vi "FusePose.vi"(0 "LIDAR range deltaX":dbl, 1 "LIDAR range deltaY":dbl, 2 "LimeLight PnP deltaX":dbl, 3 "LimeLight PnP deltaY":dbl, 4 "LimeLight range deltaX":dbl, 5 "LimeLight range deltaY":dbl, 6 "Odometry deltaY":dbl, 8 "Odometry deltaX":dbl) -> (14 "Fused deltaX":dbl, 19 "Fused deltaY":dbl)   [LabVIEW 2019]
doc: "This VI fuses multiple sensing modalities to estimate the robot's current pose."
uses:
  <vilib>/Rock Robotics/WPI/DriverStation/WPI_DriverStationRobotMode2.ctl
  sensors.vi
  dsdata.vi
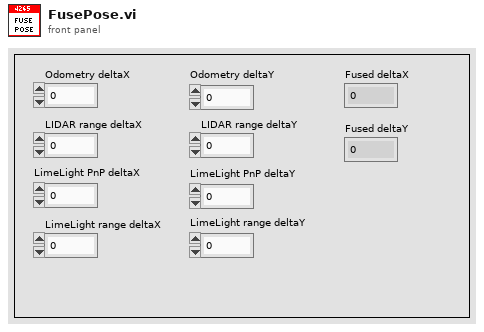
[diagram p1: front panel]
types:
  T1 = typedef "WPI_DriverStationRobotMode2.ctl" = enum16{"Autonomous Disabled", "Autonomous Enabled", "Teleop Disabled", "Teleop Enabled", "Disconnected", "Finish", "Test Disabled", "Test Enabled", "Emergency Stopped"}
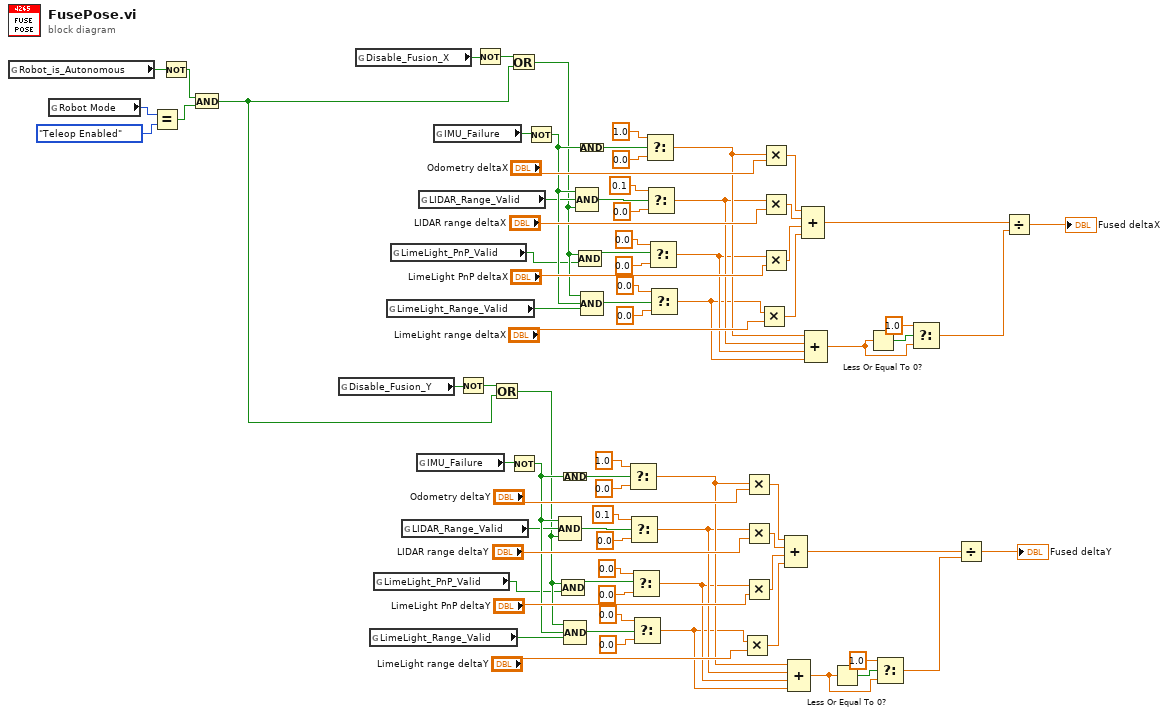
[diagram p0: block diagram]
diagram:
  n1 = global read "dsdata.vi" "Robot_is_Autonomous"() -> (w55:bool)
  n2 = global read "dsdata.vi" "Robot Mode"() -> (w54:T1)
  n3 = Equal?(x=w54, y=WPI_DriverStationRobotMode2."Teleop Enabled") -> (x = y?=w53:bool)
  n4 = Not(x=w55) -> (.not. x?=w52:bool)
  n5 = And(x=w52, y=w53) -> (x .and. y?=w9:bool)
  n6 = global read "dsdata.vi" "Disable_Fusion_Y"() -> (w16:bool)
  n7 = global read "dsdata.vi" "Disable_Fusion_X"() -> (w50:bool)
  n8 = global read "sensors.vi" "LimeLight_Range_Valid"() -> (w11:bool)
  n9 = global read "sensors.vi" "LimeLight_PnP_Valid"() -> (w12:bool)
  n10 = global read "sensors.vi" "LimeLight_Range_Valid"() -> (w45:bool)
  n11 = global read "sensors.vi" "LimeLight_PnP_Valid"() -> (w46:bool)
  n12 = global read "sensors.vi" "LIDAR_Range_Valid"() -> (w17:bool)
  n13 = global read "sensors.vi" "IMU_Failure"() -> (w22:bool)
  n14 = global read "sensors.vi" "LIDAR_Range_Valid"() -> (w56:bool)
  n15 = global read "sensors.vi" "IMU_Failure"() -> (w61:bool)
  n16 = Not(x=w16) -> (.not. x?=w15:bool)
  n17 = Not(x=w50) -> (.not. x?=w49:bool)
  n18 = Or(x=w15, y=w9) -> (x .or. y?=w13:bool)
  n19 = Or(x=w49, y=w9) -> (x .or. y?=w47:bool)
  n20 = Not(x=w22) -> (.not. x?=w20:bool)
  n21 = Not(x=w61) -> (.not. x?=w59:bool)
  n22 = Compound Arithmetic op=AND(w20, w17, w13) -> (w18:bool)
  n23 = Compound Arithmetic op=AND(w13, w12) -> (w14:bool)
  n24 = Compound Arithmetic op=AND(w20) -> (w21:bool)
  n25 = Compound Arithmetic op=AND(w13, w20, w11) -> (w19:bool)
  n26 = Compound Arithmetic op=AND(w59, w56, w47) -> (w57:bool)
  n27 = Compound Arithmetic op=AND(w47, w46) -> (w48:bool)
  n28 = Compound Arithmetic op=AND(w59) -> (w60:bool)
  n29 = Compound Arithmetic op=AND(w47, w59, w45) -> (w58:bool)
  n30 = Select(t=1.0, s=w21, f=0.0) -> (s? t:f=w26:dbl)
  n31 = Select(t=0.1, s=w18, f=0.0) -> (s? t:f=w25:dbl)
  n32 = Select(t=0.0, s=w14, f=0.0) -> (s? t:f=w24:dbl)
  n33 = Select(t=0.0, s=w19, f=0.0) -> (s? t:f=w23:dbl)
  n34 = Select(t=1.0, s=w60, f=0.0) -> (s? t:f=w65:dbl)
  n35 = Select(t=0.1, s=w57, f=0.0) -> (s? t:f=w64:dbl)
  n36 = Select(t=0.0, s=w48, f=0.0) -> (s? t:f=w63:dbl)
  n37 = Select(t=0.0, s=w58, f=0.0) -> (s? t:f=w62:dbl)
  n38 = Multiply(x=w23, y="LimeLight range deltaY") -> (x*y=w27:dbl)
  n39 = Multiply(x=w26, y="Odometry deltaY") -> (x*y=w37:dbl)
  n40 = Multiply(x=w25, y="LIDAR range deltaY") -> (x*y=w35:dbl)
  n41 = Multiply(x=w24, y="LimeLight PnP deltaY") -> (x*y=w31:dbl)
  n42 = Multiply(x=w62, y="LimeLight range deltaX") -> (x*y=w66:dbl)
  n43 = Multiply(x=w65, y="Odometry deltaX") -> (x*y=w76:dbl)
  n44 = Multiply(x=w64, y="LIDAR range deltaX") -> (x*y=w74:dbl)
  n45 = Multiply(x=w63, y="LimeLight PnP deltaX") -> (x*y=w70:dbl)
  n46 = Compound Arithmetic op=ADD(w37, w35, w31, w27) -> (w43:dbl)
  n47 = Compound Arithmetic op=ADD(w26, w25, w24, w23) -> (w2:dbl)
  n48 = Compound Arithmetic op=ADD(w76, w74, w70, w66) -> (w82:dbl)
  n49 = Compound Arithmetic op=ADD(w65, w64, w63, w62) -> (w6:dbl)
  n50 = Less Or Equal To 0?(x=w2) -> (x <= 0?=w4:bool)
  n51 = Less Or Equal To 0?(x=w6) -> (x <= 0?=w8:bool)
  n52 = Select(t=1.0, s=w4, f=w2) -> (s? t:f=w1:dbl)
  n53 = Select(t=1.0, s=w8, f=w6) -> (s? t:f=w5:dbl)
  n54 = Divide(x=w43, y=w1) -> (x/y=→"Fused deltaY":dbl)
  n55 = Divide(x=w82, y=w5) -> (x/y=→"Fused deltaX":dbl)
